vi "Layercoincidence.vi"(4 "Coincidence result queue overflow ref":refnum<vi>, 8 "error in (no error)":errorcluster, 9 "Type":T1(ring)) -> (0 "error out":errorcluster)   [LabVIEW 2016]
uses:
  Typedefs/Primary channel coincidence hunt.ctl
  Typedefs/Coincidence.ctl
  Typedefs/CoincidencesToSave.ctl
  Typedefs/CoincidenceWithGPSformat.ctl
  Global Variables/Scintillator IDs.vi
  Global Variables/Global Resolution.vi
  Global Variables/System info.vi
  Global Variables/Coincidence Windows.vi
panel:
  out "notifier out":refnum<notifier>
  out "CoincSave":refnum<queue>
  out "CoincStats":refnum<queue>
  out "StopNotifier":refnum<notifier>
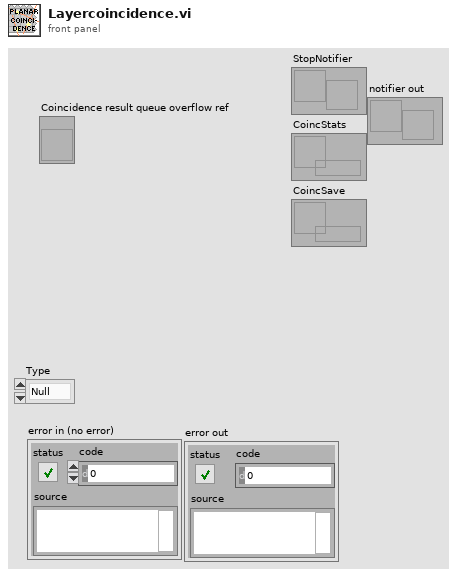
[diagram p1: front panel]
types:
  T1 = enum16{"Null", "BottomLayer", "TopAndBottom", "TopLayer"}
  T2 = cluster{"ID":i8, "NumofHits":i32, "Hits":cluster{"Time":u64, "Counted as coincidence":bool, "Coincides with":cluster{"ID":i8, "Time":u64}[]}[]}
  T3 = typedef "CoincidencesToSave.ctl" = T4[]
  T4 = typedef "CoincidenceWithGPSformat.ctl" = cluster{"Low-res hit time":u32, "Hi-res hit time":u32, "Secondary ID":i8, "DeltaT":i32, "Primary ID":i8}
  T5 = typedef "Primary channel coincidence hunt.ctl" = cluster{"Coincidences":T6[], "Secondary hits sorted":cluster{"ID":i8, "Non-coinc":u64[], "Coinc":u64[]}[], "Primary hits sorted":cluster{"ID":i8, "Non-coinc":u64[], "Coinc":u64[]}[]}
  T6 = typedef "Coincidence.ctl" = cluster{"Primary ID":i8, "Muon hit time":u64, "Secondary ID":i8, "DeltaT":i32}
  T7 = cluster{"Primary ID":i8, "Leftovers":cluster{"ID":i8, "NumofHits":i32, "Hits":cluster{"Time":u64, "Counted as coincidence":bool, "Coincides with":cluster{"ID":i8, "Time":u64}[]}[]}[]}
  T8 = cluster{"ID":i8, "NumofHits":i32, "Hits":cluster{"Time":u64, "Counted as coincidence":bool, "Coincides with":cluster{"ID":i8, "Time":u64}[]}[]}[]
  T9 = cluster{"ID":i8, "Non-coinc":i64[], "Coinc":i64[]}
  T10 = cluster{"ID":i8, "Non-coinc":u64[], "Coinc":u64[]}
  T11 = cluster{"Time":u64, "Counted as coincidence":bool, "Coincides with":cluster{"ID":i8, "Time":u64}[]}[]
  T12 = cluster{"ID":i8, "Non-coinc":u64[], "Coinc":u64[]}[]
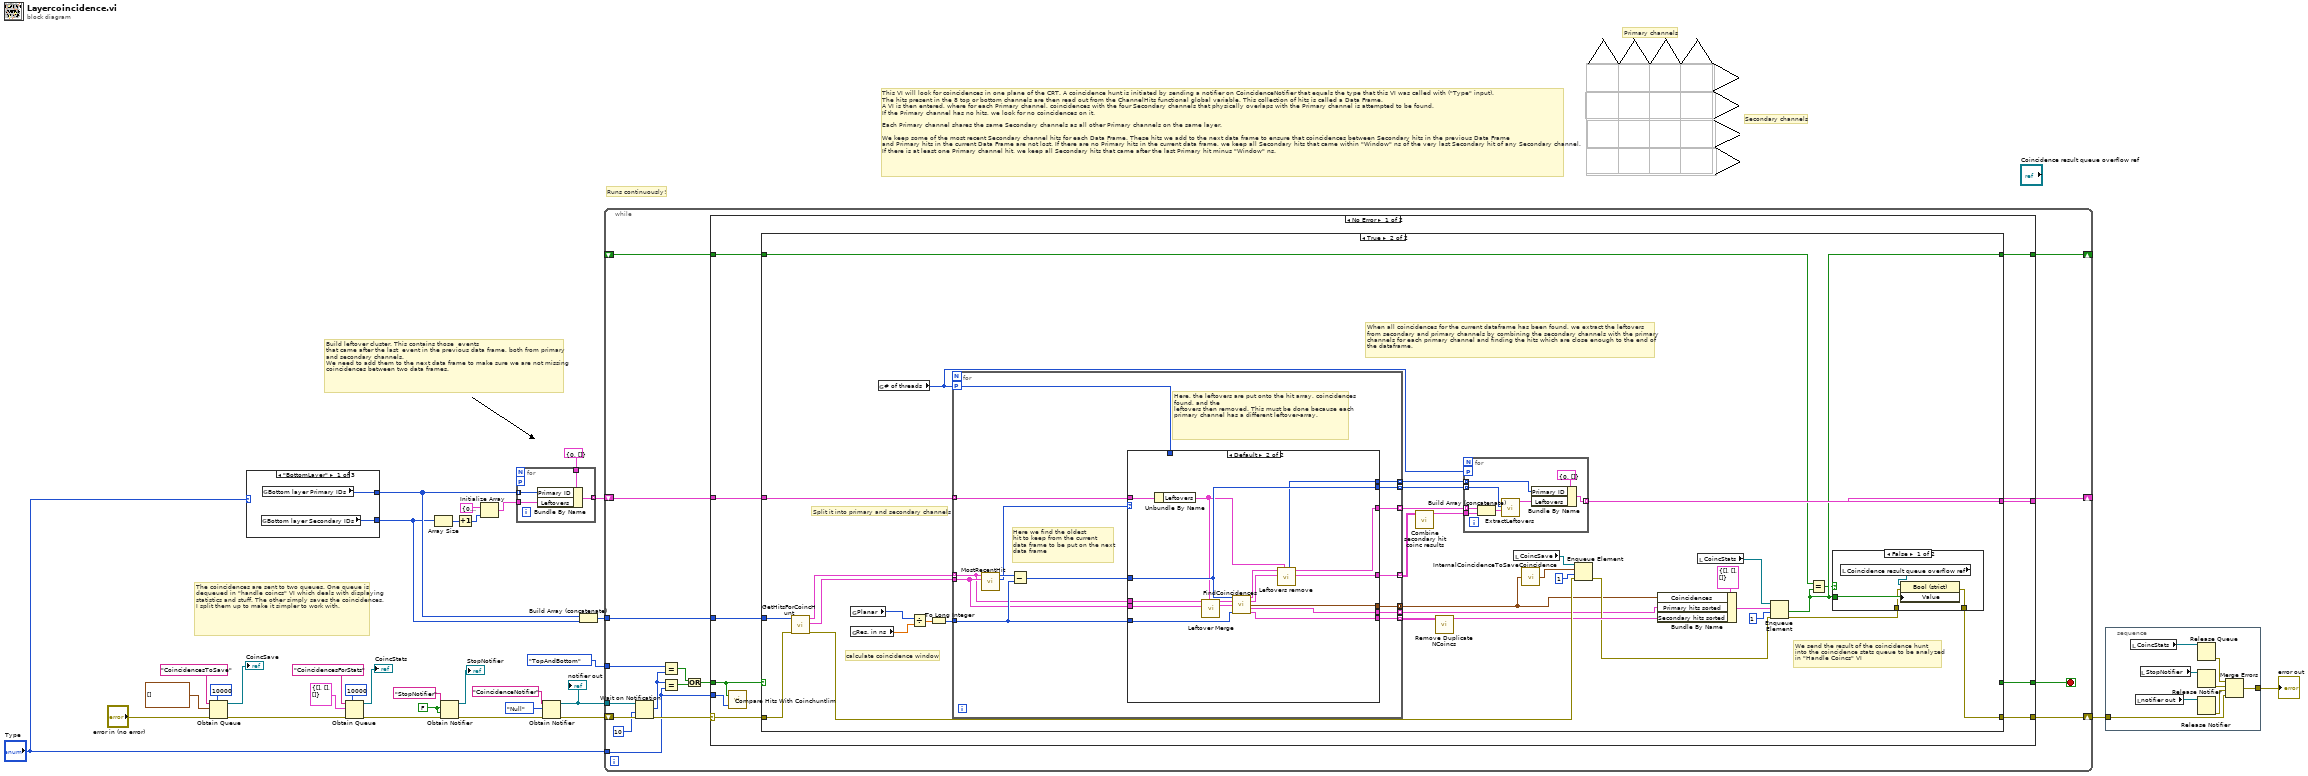
[diagram p0: block diagram]
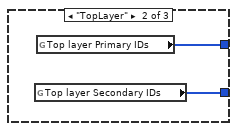
[diagram p2: hidden frame]
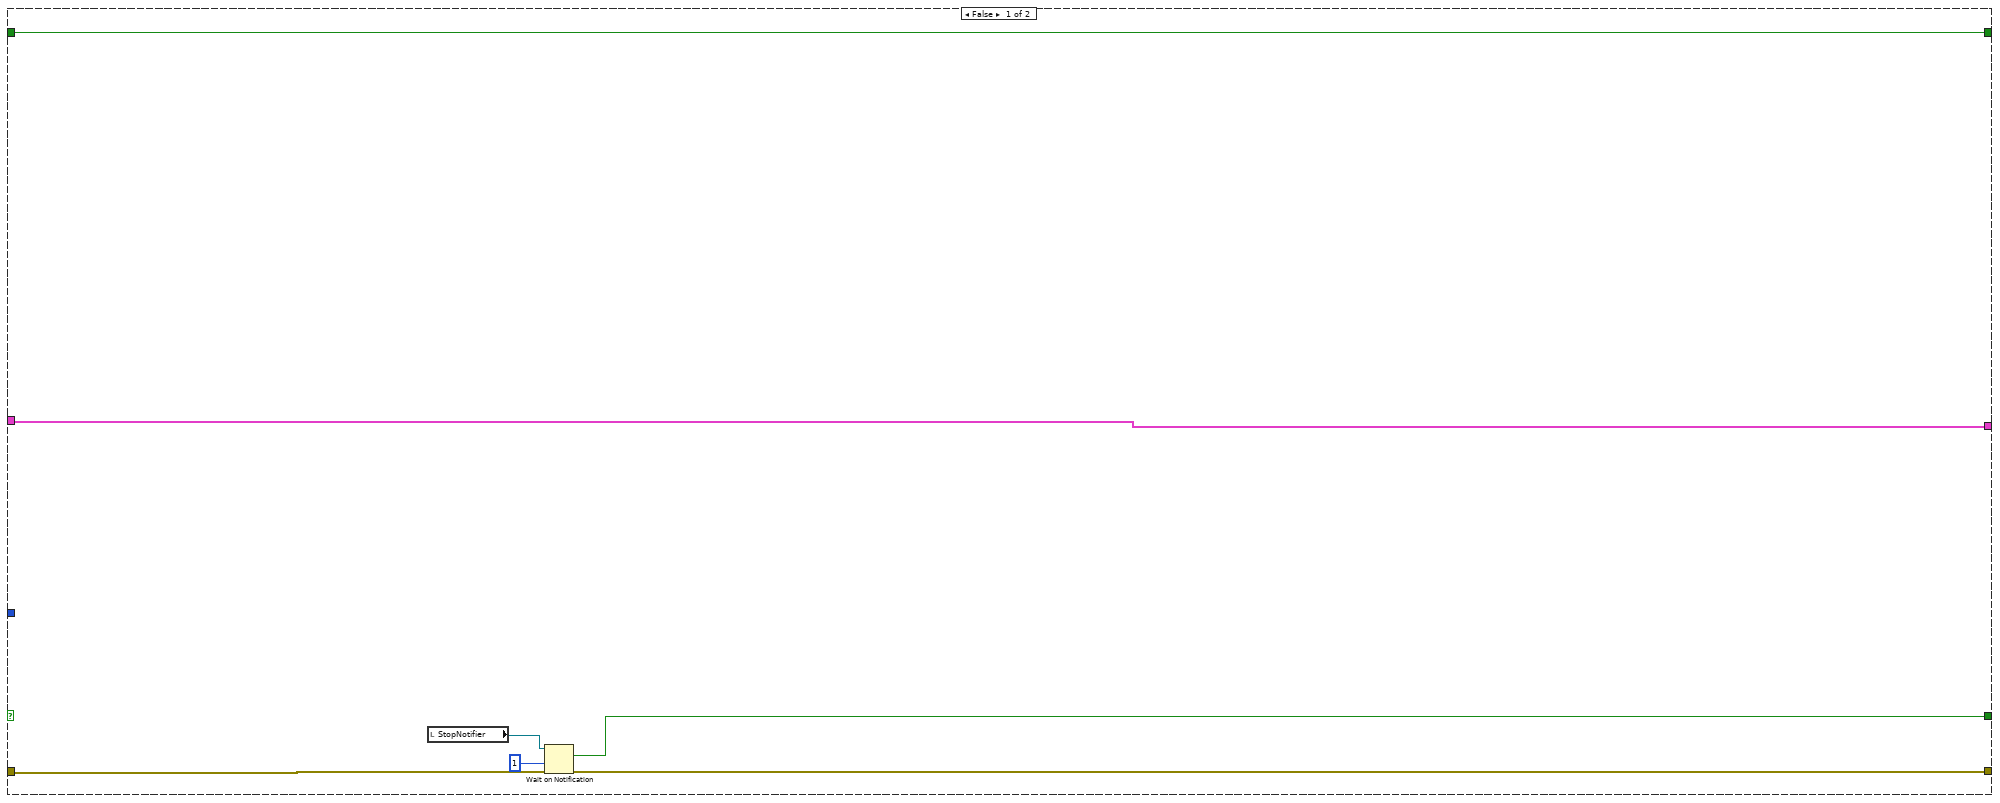
[diagram p4: hidden frame]
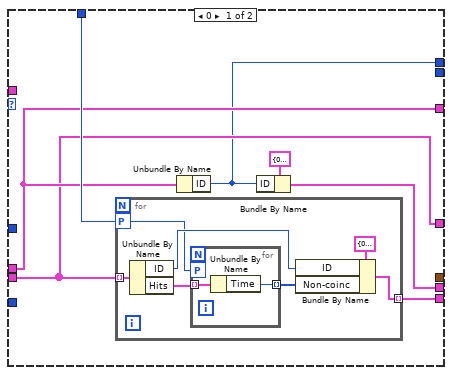
[diagram p6: hidden frame]
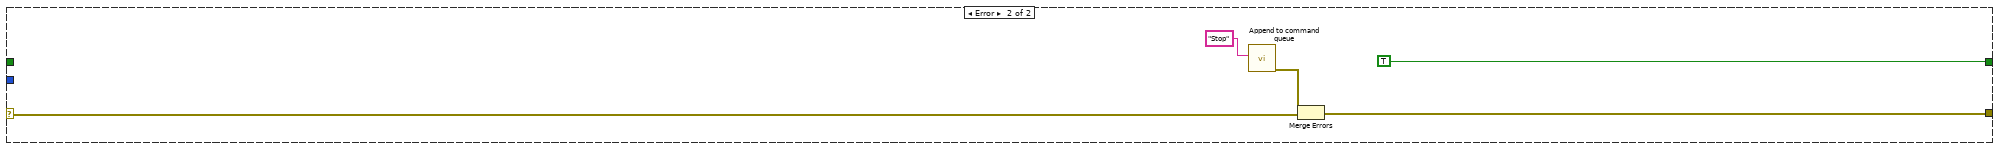
[diagram p7: hidden frame]
diagram:
  w29 = FALSE
  # "The coincidences are sent to two queues. One queue is dequeued in \"handle coincs\" VI which deals with displaying statistics and stuff. The other simply saves the coincidences. I split them up to make it simpler to work with."
  # "Runs continuously!"
  # "Secondary channels"
  # "Primary channels"
  # "This VI will look for coincidences in one plane of the CRT. A coincidence hunt is initiated by sending a notifier on CoincidenceNotifier that equals the type that this VI was called with (\"Type\" input).\nThe hits present in the 8 top or bottom channels are then read out from the ChannelHits functional global variable. This collection of hits is called a Data Frame.\nA VI is then entered, where for each Primary channel, coincidences with the four Secondary channels that physically overlaps with the Primary channel is attempted to be found. \nIf the Primary channel has no hits, we look for no coincidences on it.\n\nEach Primary channel shares the same Secondary channels as all other Primary channels on the same layer. \n\nWe keep some of the most recent Secondary channel hits for each Data Frame. These hits we add to the next data frame to ensure that coincidences between Secondary hits in the previous Data Frame\nand Primary hits in the current Data Frame are not lost. If there are no Primary hits in the current data frame, we keep all Secondary hits that came within \"Window\" ns of the very last Secondary hit of any Secondary channel. \nIf there is at least one Primary channel hit, we keep all Secondary hits that came after the last Primary hit minus \"Window\" ns."
  # "Build leftover cluster. This contains those  events \nthat came after the last  event in the previous data frame, both from primary\nand secondary channels.\nWe need to add them to the next data frame to make sure we are not missing\ncoincidences between two data frames."
  n1 = Obtain Queue(max queue size (-1, unlimited)=10000, name (unnamed)="CoincidencesToSave", element data type=T3 [] ("Coincidences"), error in (no error)="error in (no error)") -> (queue out=→"CoincSave":refnum<queue>, error out=w8:errorcluster)  [unwired: 1 in, 1 out]
  n2 = case shown="\"BottomLayer\"" "Type" {
    tunnel: [w34 w36 _] -> w5
    tunnel: [w33 w35 _] -> w4
    frame "BottomLayer" {
      n3 = global read "Scintillator IDs.vi" "Bottom layer Secondary IDs"() -> (w33:i8[])
      n4 = global read "Scintillator IDs.vi" "Bottom layer Primary IDs"() -> (w34:i8[])
    }
    frame "TopLayer" {
      n5 = global read "Scintillator IDs.vi" "Top layer Secondary IDs"() -> (w35:i8[])
      n6 = global read "Scintillator IDs.vi" "Top layer Primary IDs"() -> (w36:i8[])
    }
    frame Default {
    }
  }
  n7 = Obtain Queue(max queue size (-1, unlimited)=10000, name (unnamed)="CoincidencesForStats", element data type=T5 {"Coincidences"=[], "Secondary hits sorted"=[], "Primary hits sorted"=[]} ("Planar coincidence hunt result"), error in (no error)=w8) -> (queue out=→"CoincStats":refnum<queue>, error out=w21:errorcluster)  [unwired: 1 in, 1 out]
  n8 = Array Size(array=w4) -> (size(s)=w16:i32)
  n9 = Obtain Notifier(name (unnamed)="StopNotifier", notification data type=w29, create if not found? (T)=w29, error in (no error)=w21) -> (notifier out=→"StopNotifier":refnum<notifier>, error out=w24:errorcluster)  [unwired: 1 out]
  n10 = Increment(x=w16) -> (x+1=w15:i32)
  n11 = Initialize Array(T2 {"ID"=0, "NumofHits"=0, "Hits"=[]}, w15) -> (w30:T8)
  n12 = for {
    tunnel: T7 {"Primary ID"=0, "Leftovers"=[]} -> [w40]
    tunnel: w5 -> [w39] mode=indexing
    tunnel: [w38] -> w31 mode=indexing
    tunnel: w30 -> [w37]
    workers-P: _ -> [_]
    n13 = Bundle By Name(cluster=w40, "Primary ID"=w39, "Leftovers"=w37) -> (w38:T7)
  }
  n14 = Obtain Notifier(name (unnamed)="CoincidenceNotifier", notification data type=T1."Null" ("notification"), error in (no error)=w24) -> (notifier out=w26:refnum<notifier>, error out=w25:errorcluster)  [unwired: 1 in, 1 out]
  "notifier out" <- w26
  n15 = Build Array (concatenate)(w5, w4) -> (w14:i8[])
  n16 = while {
    tunnel: w14 -> [w56]
    shift-right: [w55] -> _
    shift-left: w31 -> [w57]
    shift-right: [w50] -> w20
    shift-left: w25 -> [w53]
    tunnel: "Type" -> [w44]
    shift-right: [w45] -> _
    shift-left: _ -> [w46]
    tunnel: w26 -> [w54]
    tunnel: T1."TopAndBottom" ("notification") -> [w42]
    stop <- w51 stop-if-true
    n17 = Wait on Notification(notifier=w54, timeout in ms (-1)=10, error in (no error)=w53) -> (notification=w41:T1, error out=w49:errorcluster)  [unwired: 1 in, 2 out]
    n18 = Equal?(x=w42, y=w41) -> (x = y?=w43:bool)
    n19 = Equal?(x=w41, y=w44) -> (x = y?=w48:bool)
    n20 = Or(x=w43, y=w48) -> (x .or. y?=w47:bool)
    n21 = case shown="No Error" w49 {
      selector: w49 -> [w63 w170]
      tunnel: w57 -> [w67 _]
      tunnel: w56 -> [w62 _]
      tunnel: [w66 _] -> w55
      tunnel: w47 -> [w58 _]
      tunnel: [w65 TRUE] -> w51
      tunnel: [w64 w172] -> w50
      tunnel: w46 -> [w61 _]
      tunnel: [w60 _] -> w45
      tunnel: w44 -> [w59 _]
      frame No Error {
        n22 = call "Compare Hits With Coinchuntlim.vi"("Type"=w59, "Make check"=w58) -> ()  [unwired: 1 out]
        n23 = case shown="True" w58 {
          tunnel: w67 -> [w70 w108]
          tunnel: w62 -> [_ w106]
          tunnel: [w70 w105] -> w66
          tunnel: w63 -> [w73 w107]
          tunnel: [w72 _] -> w65
          tunnel: [w71 w103] -> w64
          tunnel: w61 -> [w69 w104]
          tunnel: [w69 w102] -> w60
          frame False {
            n24 = local read "StopNotifier"() -> (w68:refnum<notifier>)
            n25 = Wait on Notification(notifier=w68, timeout in ms (-1)=1, error in (no error)=w73) -> (notification=w72:bool, error out=w71:errorcluster)  [unwired: 1 in, 2 out]
          }
          frame True {
            # "When all coincidences for the current dataframe has been found, we extract the leftovers\nfrom secondary and primary channels by combining the secondary channels with the primary\nchannels for each primary channel and finding the hits which are close enough to the end of\nthe dataframe."
            # "calculate coincidence window"
            # "We send the result of the coincidence hunt\ninto the coincidence stats queue to be analyzed\nin \"Handle Coincs\" VI"
            # "Split it into primary and secondary channels"
            n26 = call "GetHitsForCoincHunt.vi"("error in (no error)"=w107, "IDs"=w106) -> ("error out"=w101:errorcluster, "Secondary channels"=w83:T8, "Primary channels"=w84:T8)  [unwired: 7 in]
            n27 = global read "Global Resolution.vi" "Res. in ns"() -> (w87:ext)
            n28 = global read "Coincidence Windows.vi" "Planar"() -> (w77:i32)
            n29 = global read "System info.vi" "# of threads"() -> (w81:i32)
            n30 = Divide(x=w77, y=w87) -> (x/y=w91:ext)
            n31 = To Long Integer(number=w91) -> (32bit integer=w90:i32)
            n32 = for {
              tunnel: w84 -> [w125] mode=indexing
              tunnel: w108 -> [w136] mode=indexing
              tunnel: [w133] -> w75 mode=concatenating
              tunnel: [w132] -> w100 mode=indexing
              tunnel: [w131] -> w95 mode=indexing
              tunnel: [w130] -> w94 mode=indexing
              tunnel: w90 -> [w129]
              tunnel: w83 -> [w126]
              tunnel: [w134] -> w86 mode=indexing
              workers-P: w81 -> [w122]
              tunnel: [w124] -> w82 mode=indexing
              tunnel: [w123] -> w80 mode=indexing
              # "Here, the leftovers are put onto the hit array, coincidences found, and the\nleftovers then removed. This must be done because each primary channel has a different leftover-array."
              # "Here we find the oldest\nhit to keep from the current\ndata frame to be put on the next\ndata frame"
              n33 = call "MostRecentHit.vi"("Secondary hits"=w126, "Primary hits"=w125) -> ("NumofHits primaries"=w127:i32, "Most recent hit"=w128:u64)  [unwired: 8 in]
              n34 = Subtract(x=w128, y=w129) -> (x-y=w135:u64)
              n35 = case shown="Default" w127 {
                tunnel: w136 -> [_ w168]
                tunnel: w135 -> [_ w167]
                tunnel: [w138 w155] -> w134
                tunnel: [_ w165] -> w133
                tunnel: [w142 w166] -> w132
                tunnel: [w139 w156] -> w131
                tunnel: [_ w167] -> w130
                tunnel: w129 -> [_ w160]
                tunnel: w126 -> [w138 w164]
                tunnel: w125 -> [w139 w163]
                tunnel: [w140 w159] -> w124
                tunnel: [w137 w154] -> w123
                tunnel: w122 -> [w141 _]
                frame 0 {
                  n36 = for {
                    tunnel: [w150] -> w142 mode=indexing
                    tunnel: w138 -> [w148] mode=indexing
                    workers-P: w141 -> [w144]
                    n37 = Unbundle By Name(w148) -> ("ID"=w145:i8, "Hits"=w149:T11)
                    n38 = for {
                      tunnel: w149 -> [w151] mode=indexing
                      tunnel: [w152] -> w147 mode=indexing
                      workers-P: w144 -> [_]
                      n39 = Unbundle By Name(w151) -> ("Time"=w152:u64)
                    }
                    n40 = Bundle By Name(cluster=T10 {"ID"=0, "Non-coinc"=[], "Coinc"=[]}, "ID"=w145, "Non-coinc"=w147) -> (w150:T10)
                  }
                  n41 = Unbundle By Name(w139) -> ("ID"=w137:i8)
                  n42 = Bundle By Name(cluster=T9 {"ID"=0, "Non-coinc"=[], "Coinc"=[]} ("Primary hits sorted"), "ID"=w137) -> (w140:T9)
                }
                frame Default {
                  n43 = Unbundle By Name(w168) -> ("Leftovers"=w158:T8)
                  n44 = call "Leftover Merge.vi"("Leftovers"=w158, "Secondary hits"=w164, "Primary hits"=w163) -> ("Secondary hits out"=w161:T8, "Primary hits out"=w162:T2)  [unwired: 7 in]
                  n45 = call "FindCoincidences.vi"("Leftover candidates time"=w167, "Primary hits"=w162, "Secondary hits"=w161, "Window"=w160) -> ("Primary hits out"=w157:T2, "Secondary hits out"=w153:T8, "Coincidences"=w165:T6[], "Primary hits sorted"=w159:T10, "Secondary hits sorted"=w166:T12)  [unwired: 7 in]
                  n46 = call "Leftovers remove.vi"("Leftovers"=w158, "Secondary hits in"=w153, "Primary hits in"=w157) -> ("Secondary hits out"=w155:T8, "Primary hits out"=w156:T2, "Primary ID"=w154:i8)  [unwired: 6 in]
                }
              }
            }
            n47 = call "Combine secondary hit coinc results.vi"("secondary hits array"=w86) -> ("Combined secondaries"=w85:T8)  [unwired: 10 in]
            n48 = call "Remove Duplicate NCoincs.vi"("Secondary hits sorted"=w100) -> ("Combined"=w98:T12)  [unwired: 10 in]
            n49 = for {
              tunnel: w85 -> [w121]
              tunnel: w95 -> [w116] mode=indexing
              tunnel: w94 -> [w119] mode=indexing
              tunnel: [w117] -> w105 mode=indexing
              workers-P: w81 -> [_]
              tunnel: w80 -> [w114] mode=indexing
              n50 = Build Array (concatenate)(w116, w121) -> (w120:T8)
              n51 = call "ExtractLeftovers.vi"("Hits"=w120, "Oldest allowable hit"=w119) -> ("Leftovers new"=w118:T8)  [unwired: 9 in]
              n52 = Bundle By Name(cluster=T7 {"Primary ID"=0, "Leftovers"=[]}, "Primary ID"=w114, "Leftovers"=w118) -> (w117:T7)
            }
            n53 = local read "CoincSave"() -> (w79:refnum<queue>)
            n54 = call "InternalCoincidenceToSaveCoincidence.vi"("Coincidences"=w75) -> ("Array"=w76:T4[])
            n55 = Enqueue Element(queue=w79, element=w76, timeout in ms (-1)=1, error in (no error)=w101) -> (error out=w88:errorcluster)  [unwired: 2 out]
            n56 = Bundle By Name(cluster=T5 {"Coincidences"=[], "Secondary hits sorted"=[], "Primary hits sorted"=[]} ("Planar coincidence hunt result"), "Coincidences"=w75, "Primary hits sorted"=w82, "Secondary hits sorted"=w98) -> (w97:T5)
            n57 = local read "CoincStats"() -> (w89:refnum<queue>)
            n58 = Enqueue Element(queue=w89, element=w97, timeout in ms (-1)=1, error in (no error)=w88) -> (timed out?=w102:bool, error out=w92:errorcluster)  [unwired: 1 out]
            n59 = Equal?(x=w104, y=w102) -> (x = y?=w93:bool)
            n60 = case shown="False" w93 {
              tunnel: w102 -> [w112 _]
              tunnel: w92 -> [w111 w113]
              tunnel: [w110 w113] -> w103
              frame False {
                n61 = local read "Coincidence result queue overflow ref"() -> (w109:refnum<vi>)
                n62 = property class="Bool (strict)"(reference=w109, error in=w111, "Value"=w112) -> (error out=w110:errorcluster)  [unwired: 1 out]
              }
              frame True {
              }
            }
          }
        }
      }
      frame Error {
        n63 = call "Append to command queue.vi"("Single command"="Stop") -> ("error out"=w171:errorcluster)  [unwired: 10 in]
        n64 = Merge Errors(w171, w170) -> (w172:errorcluster)
      }
    }
  }
  n65 = stacked-sequence {
    tunnel: w20 -> [w178]
    tunnel: [w177] -> w19
    frame #0 {
      n66 = local read "CoincStats"() -> (w176:refnum<queue>)
      n67 = local read "notifier out"() -> (w174:refnum<notifier>)
      n68 = local read "StopNotifier"() -> (w175:refnum<notifier>)
      n69 = Release Queue(queue=w176) -> (error out=w181:errorcluster)  [unwired: 2 in, 2 out]
      n70 = Release Notifier(notifier=w175) -> (error out=w180:errorcluster)  [unwired: 2 in, 2 out]
      n71 = Release Notifier(notifier=w174) -> (error out=w179:errorcluster)  [unwired: 2 in, 2 out]
      n72 = Merge Errors(w181, w180, w179, w178) -> (w177:errorcluster)
    }
  }
  "error out" <- w19
